vi "PXI4072 NI-DMM Smoke Test.vi"(8 "error in (no error)":errorcluster, 11 "Instrument Descriptor":refnum<k15>) -> (0 "error out":errorcluster, 3 "Measurement":dbl format="%.5f")   [LabVIEW 2026]
uses:
  <instrlib>/niDMM/nidmm.llb/niDMM Function.ctl
  <instrlib>/niDMM/nidmm.llb/niDMM Resolution in Digits.ctl
  <instrlib>/niDMM/nidmm.llb/niDMM Configure Measurement Digits.vi
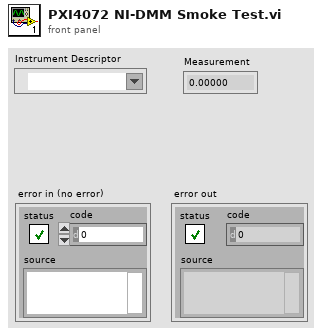
[diagram p1: front panel]
types:
  T1 = typedef "niDMM Resolution in Digits.ctl" = dbl
  T2 = typedef "niDMM Function.ctl" = enum16{"DC Volts", "AC Volts", "DC Current", "AC Current", "2-wire Resistance", "4-wire Resistance", "Diode", "Frequency", "Period", "AC Volts DC Coupled", "Capacitance", "Inductance", "Temperature"}
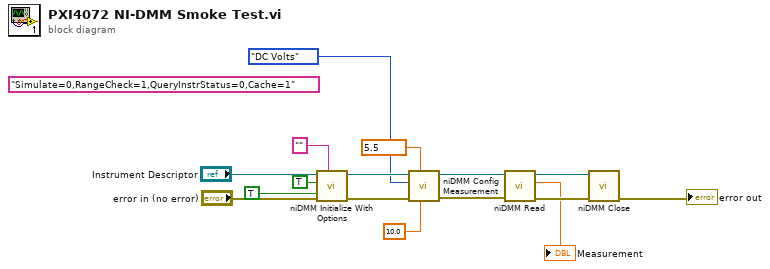
[diagram p0: block diagram]
diagram:
  w8 = T1 5.5 items=["3 1/2"=3.5, "4 1/2"=4.5, "5 1/2"=5.5, "6 1/2"=6.5, "7 1/2"=7.5] ("Resolution in Digits")
  (unwired) "Simulate=0,RangeCheck=1,QueryInstrStatus=0,Cache=1" ("Option String")
  n1 = call <instrlib>:"niDMM Initialize With Options.vi"("Option String"="", "error in (no error)"="error in (no error)", "Reset Device"=TRUE ("Reset"), "ID Query"=TRUE, "Instrument Descriptor"="Instrument Descriptor") -> ("error out"=w15:errorcluster, "instrument handle out"=w14:refnum<k15>)  [unwired: 5 in]
  n2 = call-poly <instrlib>:"niDMM Config Measurement.vi"("Range"=10.0, "Resolution in Digits"=w8, "error in (no error)"=w15, "Function"=niDMM_Function."DC Volts", "instrument handle"=w14) -> ("error out"=w6:errorcluster, "instrument handle out"=w7:refnum<k15>)  [unwired: 5 in]
  n3 = call <instrlib>:"niDMM Read.vi"("error in (no error)"=w6, "instrument handle"=w7) -> ("error out"=w5:errorcluster, "Measurement"=→"Measurement":dbl, "instrument handle out"=w3:refnum<k15>)  [unwired: 7 in]
  n4 = call <instrlib>:"niDMM Close.vi"("error in (no error)"=w5, "instrument handle"=w3) -> ("error out"=→"error out":errorcluster)  [unwired: 9 in]
